vi "FRCts20_WebMethods_Search_GET.vi"(11 "httpRequestID":u32) -> ()   [LabVIEW 2014, in "FRCts20_WebMethods.lvlib"]
uses:
  FRCts20_WebMethods.lvlib
  <vilib>/wsapi/NI_WebServices.lvlib
  Backend/source/VI Source/FRCts20_Backend_API/FRCts20_Backend_API_Team.vi
  Backend/source/VI Source/FRCts20_Backend_API/FRCts20_Backend_API_Command_Team.ctl
  Backend/source/VI Source/FRCts20_Backend_API/FRCts20_Backend_API_SW.ctl
  Backend/source/VI Source/FRCts20_Backend_API/FRCts20_Backend_API_Status.ctl
  Backend/source/VI Source/FRCts20_Backend_API/FRCts20_Backend_API_Team.ctl
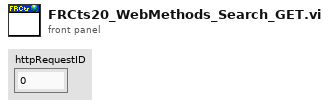
[diagram p1: front panel]
types:
  T1 = typedef "FRCts20_Backend_API.lvlib/FRCts20_Backend_API_Command_Team.ctl" = string
  T2 = typedef "FRCts20_Backend_API.lvlib/FRCts20_Backend_API_Team.ctl" = cluster{"Team Index":u32, "Team Number":u32, "Team Name":string, "Short Team Name":string, "Nick Name":string, "Robot Name":string, "City":string, "State":string, "Country":string, "Rookie Year":u32, "SWType":T3, "CAN":bool, "Vision":bool, "Kinect":bool, "Tags":string, "Avatar":string, "Request Array":cluster{"Request Index":u32, "Description":string, "Status":T4, "Open Date":timestamp, "Last Update":timestamp, "Close Date":timestamp}[], "Events Attending":cluster{"EventIndex":dbl, "EventName":string, "IsLive":bool}[], "APIReturn":string}
  T3 = typedef "FRCts20_Backend_API.lvlib/FRCts20_Backend_API_SW.ctl" = string
  T4 = typedef "FRCts20_Backend_API.lvlib/FRCts20_Backend_API_Status.ctl" = enum16{"Open", "In Work", "Closed"}
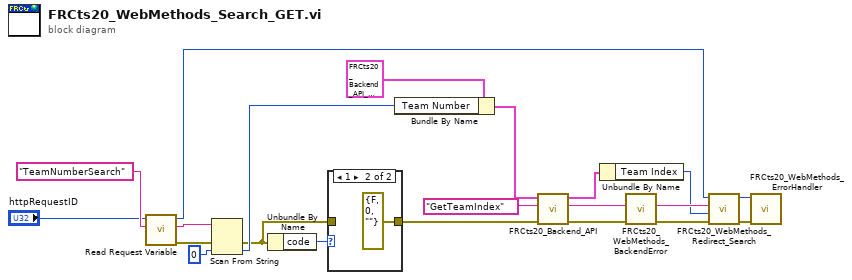
[diagram p0: block diagram]
diagram:
  n1 = call <vilib>:"Read Request Variable.vi"("variable name"="TeamNumberSearch", "httpRequestID"="httpRequestID") -> ("error out"=w11:errorcluster, "value"=w8:string, "httpRequestID out"=w12:u32)  [unwired: 7 in]
  n2 = Scan From String(input string=w8, error in=w11, default 1=u32 0 ("Team Number")) -> (error out=w4:errorcluster, output 1=w9:u32)  [unwired: 2 in, 2 out]
  n3 = Unbundle By Name(w4) -> ("code"=w5:i32)
  n4 = case shown="1" w5 {
    tunnel: [w22 errorcluster {"status"=FALSE, "code"=0, "source"=""} ("error IO")] -> w3
    tunnel: w4 -> [w22 _]
    frame 0, Default {
    }
    frame 1 {
    }
  }
  n5 = Bundle By Name(cluster=T2 {"Team Index"=0, "Team Number"=0, "Team Name"="", "Short Team Name"="", "Nick Name"="", "Robot Name"="", "City"="", "State"="", "Country"="", "Rookie Year"=0, "SWType"="", "CAN"=FALSE, "Vision"=FALSE, "Kinect"=FALSE, "Tags"="", "Avatar"="", "Request Array"=[], "Events Attending"=[], "APIReturn"=""} ("Team In"), "Team Number"=w9) -> (w15:T2)
  n6 = call-poly "FRCts20_Backend_API.vi"("error in (no error)"=w3, "Command"=T1 "GetTeamIndex", "Team In"=w15) -> ("error out"=w14:errorcluster, "Status"=w13:string, "Team Out"=w20:T2)  [unwired: 6 in]
  n7 = Unbundle By Name(w20) -> ("Team Index"=w6:u32)
  n8 = call "FRCts20_WebMethods_BackendError.vi"("error in (no error)"=w14, "Status"=w13) -> ("error out"=w19:errorcluster, "Status out"=w7:string)  [unwired: 8 in]
  n9 = call "FRCts20_WebMethods_Redirect_Search.vi"("error in (no error)"=w19, "Team Index"=w6, "Status"=w7, "httpRequestID"=w12) -> ("error out"=w18:errorcluster, "httpRequestID out"=w17:u32)  [unwired: 6 in]
  n10 = call "FRCts20_WebMethods_ErrorHandler.vi"("error in"=w18, "LabVIEW Web Service Request"=w17) -> ()  [unwired: 8 in, 2 out]
